vi "test_read-nmea-data2.vi"() -> ()   [LabVIEW 2019] (continued)
\t$GBGSV,2,2,06,33,62,220,31,34,,,33,1*41\n\t\n15:14:39.69\tF9P\t$GBGSV,1,1,03,11,48,133,,14,87,101,,33,62,220,,3*44\n\t\n15:14:39.71\tF9P\t$GNGLL,3723.60486,N,12656.97250,E,061441.00,A,A*77\n\t\n15:14:39.73\tF9P\t\t\n15:14:39.75\tF9P\t\t\n15:14:39.77\tF9P\t\t\n15:14:39.79\tF9P\t\t\n15:14:39.81\tF9P\t\t\n15:14:39.83\tF9P\t\t\n15:14:39.85\tF9P\t\t\n15:14:39.87\tF9P\t\t\n15:14:39.89\tF9P\t\t\n15:14:39.91\tF9P\t\t\n15:14:39.93\tF9P\t\t\n15:14:39.95\tF9P\t\t\n15:14:39.97\tF9P\t\t\n15:14:39.99\tF9P\t\t\n15:14:40.01\tF9P\t\t\n15:14:40.03\tF9P\t\t\n15:14:40.05\tF9P\t\t\n15:14:40.07\tF9P\t\t\n15:14:40.09\tF9P\t\t\n15:14:40.11\tF9P\t\t\n15:14:40.13\tF9P\t\t\n15:14:40.15\tF9P\t\t\n15:14:40.17\tF9P\t\t\n15:14:40.19\tF9P\t\t\n15:14:40.21\tF9P\t\t\n15:14:40.23\tF9P\t$GNRMC,061442.00,A,3723.60477,N,12656.97181,E,2.294,241.48,250720,,,A,V*0C\n\t\n15:14:40.25\tF9P\t$GNVTG,241.48,T,,M,2.294,N,4.248,K,A*2F\n\t\n15:14:40.27\tF9P\t$GNGGA,061442.00,3723.60477,N,12656.97181,E,1,12,0.66,44.9,M,18.5,M,,*76\n\t\n15:14:40.29\tF9P\t$GNGSA,A,3,12,06,19,05,17,09,04,02,,,,,1.17,0.66,0.97,1*09\n\t\n15:14:40.31\tF9P\t$GNGSA,A,3,85,70,71,84,,,,,,,,,1.17,0.66,0.97,2*0B\n\t\n15:14:40.33\tF9P\t$GNGSA,A,3,36,19,11,04,09,12,,,,,,,1.17,0.66,0.97,3*09\n\t\n15:14:40.35\tF9P\t$GNGSA,A,3,14,11,33,,,,,,,,,,1.17,0.66,0.97,4*08\n\t\n15:14:40.37\tF9P\t$GPGSV,3,1,09,02,55,320,33,04,17,043,38,05,38,248,35,06,64,050,28,1*6F\n\t\n15:14:40.39\tF9P\t$GPGSV,3,2,09,09,44,073,38,12,23,276,24,17,32,154,35,19,51,157,36,1*66\n\t\n15:14:40.41\tF9P\t$GPGSV,3,3,09,25,12,306,18,1*55\n\t\n15:14:40.43\tF9P\t$GPGSV,3,1,09,02,55,320,,04,17,043,26,05,38,248,25,06,64,050,24,6*6A\n\t\n15:14:40.45\tF9P\t$GPGSV,3,2,09,09,44,073,25,12,23,276,15,17,32,154,20,19,51,157,,6*6E\n\t\n15:14:40.47\tF9P\t$GPGSV,3,3,09,25,12,306,,6*5B\n\t\n15:14:40.49\tF9P\t$GLGSV,2,1,08,69,10,031,27,70,70,037,26,71,54,207,31,72,05,210,,1*79\n\t\n15:14:40.51\tF9P\t$GLGSV,2,2,08,77,01,324,,84,19,123,20,85,69,072,37,86,38,331,,1*75\n\t\n15:14:40.53\tF9P\t$GLGSV,2,1,08,69,10,031,21,70,70,037,,71,54,207,30,72,05,210,,3*78\n\t\n15:14:40.55\tF9P\t$GLGSV,2,2,08,77,01,324,,84,19,123,26,85,69,072,24,86,38,331,,3*73\n\t\n15:14:40.57\tF9P\t$GAGSV,2,1,08,02,08,296,11,04,67,115,24,09,33,193,27,11,72,001,24,7*7C\n\t\n15:14:40.59\tF9P\t$GAGSV,2,2,08,12,39,103,30,19,25,045,28,25,08,248,,36,27,309,19,7*74\n\t\n15:14:40.61\tF9P\t$GAGSV,2,1,08,02,08,296,,04,67,115,,09,33,193,,11,72,001,,2*7C\n\t\n15:14:40.63\tF9P\t$GAGSV,2,2,08,12,39,103,,19,25,045,,25,08,248,,36,27,309,,2*70\n\t\n15:14:40.65\tF9P\t$GBGSV,2,1,06,07,,,24,11,48,133,28,14,87,101,31,28,,,24,1*71\n\t\n15:14:40.67\tF9P\t$GBGSV,2,2,06,33,62,220,37,34,,,37,1*43\n\t\n15:14:40.69\tF9P\t$GBGSV,1,1,03,11,48,133,22,14,87,101,,33,62,220,,3*44\n\t\n15:14:40.71\tF9P\t$GNGLL,3723.60477,N,12656.97181,E,061442.00,A,A*75\n\t\n15:14:40.73\tF9P\t\t\n15:14:40.75\tF9P\t\t\n15:14:40.77\tF9P\t\t\n15:14:40.79\tF9P\t\t\n15:14:40.81\tF9P\t\t\n15:14:40.83\tF9P\t\t\n15:14:40.85\tF9P\t\t\n15:14:40.87\tF9P\t\t\n15:14:40.89\tF9P\t\t\n15:14:40.91\tF9P\t\t\n15:14:40.93\tF9P\t\t\n15:14:40.95\tF9P\t\t\n15:14:40.97\tF9P\t\t\n15:14:40.99\tF9P\t\t\n15:14:41.01\tF9P\t\t\n15:14:41.03\tF9P\t\t\n15:14:41.05\tF9P\t\t\n15:14:41.07\tF9P\t\t\n15:14:41.09\tF9P\t\t\n15:14:41.11\tF9P\t\t\n15:14:41.13\tF9P\t\t\n15:14:41.15\tF9P\t\t\n15:14:41.17\tF9P\t\t\n15:14:41.19\tF9P\t\t\n15:14:41.21\tF9P\t\t\n15:14:41.23\tF9P\t$GNRMC,061443.00,A,3723.60479,N,12656.97102,E,2.245,246.31,250720,,,A,V*0D\n\t\n15:14:41.25\tF9P\t$GNVTG,246.31,T,,M,2.245,N,4.157,K,A*27\n\t\n15:14:41.27\tF9P\t$GNGGA,061443.00,3723.60479,N,12656.97102,E,1,12,0.63,45.0,M,18.5,M,,*7F\n\t\n15:14:41.29\tF9P\t$GNGSA,A,3,12,06,19,05,17,09,04,02,,,,,1.14,0.63,0.95,1*0D\n\t\n15:14:41.31\tF9P\t$GNGSA,A,3,85,70,71,84,,,,,,,,,1.14,0.63,0.95,2*0F\n\t\n15:14:41.33\tF9P\t$GNGSA,A,3,36,19,11,04,09,12,,,,,,,1.14,0.63,0.95,3*0D\n\t\n15:14:41.35\tF9P\t$GNGSA,A,3,14,11,33,,,,,,,,,,1.14,0.63,0.95,4*0C\n\t\n15:14:41.37\tF9P\t$GPGSV,3,1,09,02,55,320,34,04,17,043,33,05,38,248,34,06,64,050,28,1*62\n\t\n15:14:41.39\tF9P\t$GPGSV,3,2,09,09,44,073,36,12,23,276,26,17,32,154,44,19,51,157,33,1*69\n\t\n15:14:41.41\tF9P\t$GPGSV,3,3,09,25,12,306,17,1*5A\n\t\n15:14:41.43\tF9P\t$GPGSV,3,1,09,02,55,320,,04,17,043,27,05,38,248,25,06,64,050,25,6*6A\n\t\n15:14:41.45\tF9P\t$GPGSV,3,2,09,09,44,073,25,12,23,276,14,17,32,154,21,19,51,157,,6*6E\n\t\n15:14:41.47\tF9P\t$GPGSV,3,3,09,25,12,306,,6*5B\n\t\n15:14:41.49\tF9P\t$GLGSV,2,1,08,69,10,031,32,70,70,037,27,71,54,207,35,72,05,210,,1*78\n\t\n15:14:41.51\tF9P\t$GLGSV,2,2,08,77,01,324,,84,19,123,19,85,69,072,35,86,38,331,,1*7D\n\t\n15:14:41.53\tF9P\t$GLGSV,2,1,08,69,10,031,20,70,70,037,,71,54,207,20,72,05,210,,3*78\n\t\n15:14:41.55\tF9P\t$GLGSV,2,2,08,77,01,324,,84,19,123,24,85,69,072,23,86,38,331,,3*76\n\t\n15:14:41.57\tF9P\t$GAGSV,2,1,08,02,08,296,10,04,67,115,26,09,33,193,32,11,72,001,24,7*7B\n\t\n15:14:41.59\tF9P\t$GAGSV,2,2,08,12,39,103,23,19,25,045,33,25,08,248,24,36,27,309,19,7*7A\n\t\n15:14:41.61\tF9P\t$GAGSV,2,1,08,02,08,296,,04,67,115,,09,33,193,,11,72,001,,2*7C\n\t\n15:14:41.63\tF9P\t$GAGSV,2,2,08,12,39,103,,19,25,045,,25,08,248,,36,27,309,,2*70\n\t\n15:14:41.65\tF9P\t$GBGSV,2,1,06,07,,,25,11,48,133,38,14,87,101,32,28,,,24,1*72\n\t\n15:14:41.67\tF9P\t$GBGSV,2,2,06,33,62,220,26,34,,,42,1*41\n\t\n15:14:41.69\tF9P\t$GBGSV,1,1,03,11,48,133,,14,87,101,,33,62,220,,3*44\n\t\n15:14:41.71\tF9P\t$GNGLL,3723.60479,N,12656.97102,E,061443.00,A,A*71\n\t\n15:14:41.73\tF9P\t\t\n15:14:41.75\tF9P\t\t\n15:14:41.77\tF9P\t\t\n15:14:41.79\tF9P\t\t\n15:14:41.81\tF9P\t\t\n15:14:41.83\tF9P\t\t\n15:14:41.85\tF9P\t\t\n15:14:41.87\tF9P\t\t\n15:14:41.89\tF9P\t\t\n15:14:41.91\tF9P\t\t\n15:14:41.93\tF9P\t\t\n15:14:41.95\tF9P\t\t\n15:14:41.97\tF9P\t\t\n15:14:41.99\tF9P\t\t\n15:14:42.01\tF9P\t\t\n15:14:42.03\tF9P\t\t\n15:14:42.05\tF9P\t\t\n15:14:42.07\tF9P\t\t\n15:14:42.09\tF9P\t\t\n15:14:42.11\tF9P\t\t\n15:14:42.13\tF9P\t\t\n15:14:42.15\tF9P\t\t\n15:14:42.17\tF9P\t\t\n15:14:42.19\tF9P\t\t\n15:14:42.21\tF9P\t\t\n15:14:42.23\tF9P\t$GNRMC,061444.00,A,3723.60478,N,12656.97021,E,2.480,246.00,250720,,,A,V*06\n\t\n15:14:42.25\tF9P\t$GNVTG,246.00,T,,M,2.480,N,4.594,K,A*21\n\t\n15:14:42.27\tF9P\t$GNGGA,061444.00,3723.60478,N,12656.97021,E,1,12,0.63,45.2,M,18.5,M,,*7B\n\t\n15:14:42.29\tF9P\t$GNGSA,A,3,12,06,19,05,17,09,04,02,,,,,1.14,0.63,0.95,1*0D\n\t\n15:14:42.31\tF9P\t$GNGSA,A,3,85,70,71,84,,,,,,,,,1.14,0.63,0.95,2*0F\n\t\n15:14:42.33\tF9P\t$GNGSA,A,3,36,19,11,04,09,12,,,,,,,1.14,0.63,0.95,3*0D\n\t\n15:14:42.35\tF9P\t$GNGSA,A,3,14,11,33,,,,,,,,,,1.14,0.63,0.95,4*0C\n\t\n15:14:42.37\tF9P\t$GPGSV,3,1,09,02,55,320,29,04,17,043,35,05,38,248,32,06,64,050,29,1*6F\n\t\n15:14:42.39\tF9P\t$GPGSV,3,2,09,09,44,073,36,12,23,276,26,17,32,154,42,19,51,157,33,1*6F\n\t\n15:14:42.41\tF9P\t$GPGSV,3,3,09,25,12,306,17,1*5A\n\t\n15:14:42.43\tF9P\t$GPGSV,3,1,09,02,55,320,,04,17,043,26,05,38,248,24,06,64,050,27,6*68\n\t\n15:14:42.45\tF9P\t$GPGSV,3,2,09,09,44,073,25,12,23,276,17,17,32,154,23,19,51,157,,6*6F\n\t\n15:14:42.47\tF9P\t$GPGSV,3,3,09,25,12,306,,6*5B\n\t\n15:14:42.49\tF9P\t$GLGSV,2,1,08,69,10,031,33,70,70,037,27,71,54,207,34,72,05,210,,1*78\n\t\n15:14:42.51\tF9P\t$GLGSV,2,2,08,77,01,324,,84,19,123,20,85,69,072,31,86,38,331,,1*73\n\t\n15:14:42.53\tF9P\t$GLGSV,2,1,08,69,10,031,20,70,70,037,,71,54,207,22,72,05,210,,3*7A\n\t\n15:14:42.55\tF9P\t$GLGSV,2,2,08,77,01,324,,84,19,123,30,85,69,072,24,86,38,331,,3*74\n\t\n15:14:42.57\tF9P\t$GAGSV,2,1,08,02,08,296,09,04,67,115,31,09,33,193,32,11,72,001,24,7*75\n\t\n15:14:42.59\tF9P\t$GAGSV,2,2,08,12,39,103,23,19,25,045,35,25,08,248,23,36,27,309,20,7*71\n\t\n15:14:42.61\tF9P\t$GAGSV,2,1,08,02,08,296,,04,67,115,,09,33,193,,11,72,001,,2*7C\n\t\n15:14:42.63\tF9P\t$GAGSV,2,2,08,12,39,103,,19,25,045,,25,08,248,,36,27,309,,2*70\n\t\n15:14:42.65\tF9P\t$GBGSV,2,1,06,07,,,25,11,48,133,39,14,87,101,27,28,,,26,1*75\n\t\n15:14:42.67\tF9P\t$GBGSV,2,2,06,33,62,220,31,34,,,46,1*43\n\t\n15:14:42.69\tF9P\t$GBGSV,1,1,03,11,48,133,24,14,87,101,,33,62,220,,3*42\n\t\n15:14:42.71\tF9P\t$GNGLL,3723.60478,N,12656.97021,E,061444.00,A,A*77\n\t\n15:14:42.73\tF9P\t\t\n15:14:42.75\tF9P\t\t\n15:14:42.77\tF9P\t\t\n15:14:42.79\tF9P\t\t\n15:14:42.81\tF9P\t\t\n15:14:42.83\tF9P\t\t\n15:14:42.85\tF9P\t\t\n15:14:42.87\tF9P\t\t\n15:14:42.89\tF9P\t\t\n15:14:42.91\tF9P\t\t\n15:14:42.93\tF9P\t\t\n15:14:42.95\tF9P\t\t\n15:14:42.97\tF9P\t\t\n15:14:42.99\tF9P\t\t\n15:14:43.01\tF9P\t\t\n15:14:43.03\tF9P\t\t\n15:14:43.05\tF9P\t\t\n15:14:43.07\tF9P\t\t\n15:14:43.09\tF9P\t\t\n15:14:43.11\tF9P\t\t\n15:14:43.13\tF9P\t\t\n15:14:43.15\tF9P\t\t\n15:14:43.17\tF9P\t\t\n15:14:43.19\tF9P\t\t\n15:14:43.21\tF9P\t\t\n15:14:43.23\tF9P\t$GNRMC,061445.00,A,3723.60468,N,12656.96939,E,2.508,244.25,250720,,,A,V*03\n\t\n15:14:43.25\tF9P\t$GNVTG,244.25,T,,M,2.508,N,4.645,K,A*2A\n\t\n15:14:43.27\tF9P\t$GNGGA,061445.00,3723.60468,N,12656.96939,E,1,12,0.66,45.7,M,18.5,M,,*7A\n\t\n15:14:43.29\tF9P\t$GNGSA,A,3,12,06,19,05,17,09,04,02,,,,,1.17,0.66,0.97,1*09\n\t\n15:14:43.31\tF9P\t$GNGSA,A,3,85,70,71,84,,,,,,,,,1.17,0.66,0.97,2*0B\n\t\n15:14:43.33\tF9P\t$GNGSA,A,3,36,19,11,04,09,12,,,,,,,1.17,0.66,0.97,3*09\n\t\n15:14:43.35\tF9P\t$GNGSA,A,3,14,11,33,,,,,,,,,,1.17,0.66,0.97,4*08\n\t\n15:14:43.37\tF9P\t$GPGSV,3,1,09,02,55,320,30,04,17,043,35,05,38,248,35,06,64,050,36,1*6E\n\t\n15:14:43.39\tF9P\t$GPGSV,3,2,09,09,44,073,37,12,23,276,26,17,32,154,28,19,51,157,28,1*68\n\t\n15:14:43.41\tF9P\t$GPGSV,3,3,09,25,12,306,16,1*5B\n\t\n15:14:43.43\tF9P\t$GPGSV,3,1,09,02,55,320,,04,17,043,25,05,38,248,24,06,64,050,27,6*6B\n\t\n15:14:43.45\tF9P\t$GPGSV,3,2,09,09,44,073,26,12,23,276,18,17,32,154,22,19,51,157,,6*62\n\t\n15:14:43.47\tF9P\t$GPGSV,3,3,09,25,12,306,,6*5B\n\t\n15:14:43.49\tF9P\t$GLGSV,2,1,08,69,10,031,29,70,70,037,27,71,54,207,39,72,05,210,,1*7E\n\t\n15:14:43.51\tF9P\t$GLGSV,2,2,08,77,01,324,,84,19,123,21,85,69,072,34,86,38,331,,1*77\n\t\n15:14:43.53\tF9P\t$GLGSV,2,1,08,69,10,031,20,70,70,037,,71,54,207,24,72,05,210,,3*7C\n\t\n15:14:43.55\tF9P\t$GLGSV,2,2,08,77,01,324,,84,19,123,25,85,69,072,26,86,38,331,,3*72\n\t\n15:14:43.57\tF9P\t$GAGSV,2,1,08,02,08,296,09,04,67,115,33,09,33,193,26,11,72,001,24,7*72\n\t\n15:14:43.59\tF9P\t$GAGSV,2,2,08,12,39,103,31,19,25,045,26,25,08,248,21,36,27,309,20,7*72\n\t\n15:14:43.61\tF9P\t$GAGSV,2,1,08,02,08,296,,04,67,115,21,09,33,193,,11,72,001,,2*7F\n\t\n15:14:43.63\tF9P\t$GAGSV,2,2,08,12,39,103,,19,25,045,,25,08,248,,36,27,309,,2*70\n\t\n15:14:43.65\tF9P\t$GBGSV,2,1,06,07,,,25,11,48,133,39,14,87,101,27,28,,,25,1*76\n\t\n15:14:43.67\tF9P\t$GBGSV,2,2,06,33,62,220,34,34,,,37,1*40\n\t\n15:14:43.69\tF9P\t$GBGSV,1,1,03,11,48,133,26,14,87,101,29,33,62,220,,3*4B\n\t\n15:14:43.71\tF9P\t$GNGLL,3723.60468,N,12656.96939,E,061445.00,A,A*76\n\t\n15:14:43.73\tF9P\t\t\n15:14:43.75\tF9P\t\t\n15:14:43.77\tF9P\t\t\n15:14:43.79\tF9P\t\t\n15:14:43.81\tF9P\t\t\n15:14:43.83\tF9P\t\t\n15:14:43.85\tF9P\t\t\n15:14:43.87\tF9P\t\t\n15:14:43.89\tF9P\t\t\n15:14:43.91\tF9P\t\t\n15:14:43.93\tF9P\t\t\n15:14:43.95\tF9P\t\t\n15:14:43.97\tF9P\t\t\n15:14:43.99\tF9P\t\t\n15:14:44.01\tF9P\t\t\n15:14:44.03\tF9P\t\t\n15:14:44.05\tF9P\t\t\n15:14:44.07\tF9P\t\t\n15:14:44.09\tF9P\t\t\n15:14:44.11\tF9P\t\t\n15:14:44.13\tF9P\t\t\n15:14:44.15\tF9P\t\t\n15:14:44.17\tF9P\t\t\n15:14:44.19\tF9P\t\t\n15:14:44.21\tF9P\t\t\n15:14:44.23\tF9P\t$GNRMC,061446.00,A,3723.60454,N,12656.96856,E,2.232,243.16,250720,,,A,V*0E\n\t\n15:14:44.25\tF9P\t$GNVTG,243.16,T,,M,2.232,N,4.135,K,A*23\n\t\n15:14:44.27\tF9P\t$GNGGA,061446.00,3723.60454,N,12656.96856,E,1,12,0.66,45.7,M,18.5,M,,*7E\n\t\n15:14:44.29\tF9P\t$GNGSA,A,3,12,06,19,05,17,09,04,02,,,,,1.17,0.66,0.97,1*09\n\t\n15:14:44.31\tF9P\t$GNGSA,A,3,85,70,71,84,,,,,,,,,1.17,0.66,0.97,2*0B\n\t\n15:14:44.33\tF9P\t$GNGSA,A,3,36,19,11,04,09,12,,,,,,,1.17,0.66,0.97,3*09\n\t\n15:14:44.35\tF9P\t$GNGSA,A,3,14,11,33,,,,,,,,,,1.17,0.66,0.97,4*08\n\t\n15:14:44.37\tF9P\t$GPGSV,3,1,09,02,56,320,29,04,17,043,30,05,38,248,35,06,64,050,40,1*61\n\t\n15:14:44.39\tF9P\t$GPGSV,3,2,09,09,44,073,33,12,23,276,25,17,32,154,33,19,51,157,36,1*6A\n\t\n15:14:44.41\tF9P\t$GPGSV,3,3,09,25,12,306,16,1*5B\n\t\n15:14:44.43\tF9P\t$GPGSV,3,1,09,02,56,320,,04,17,043,24,05,38,248,25,06,64,050,27,6*68\n\t\n15:14:44.45\tF9P\t$GPGSV,3,2,09,09,44,073,25,12,23,276,17,17,32,154,20,19,51,157,,6*6C\n\t\n15:14:44.47\tF9P\t$GPGSV,3,3,09,25,12,306,,6*5B\n\t\n15:14:44.49\tF9P\t$GLGSV,2,1,08,69,10,031,31,70,70,037,29,71,54,207,36,72,05,210,,1*76\n\t\n15:14:44.51\tF9P\t$GLGSV,2,2,08,77,01,324,,84,19,123,22,85,69,072,28,86,38,331,,1*79\n\t\n15:14:44.53\tF9P\t$GLGSV,2,1,08,69,10,031,19,70,70,037,,71,54,207,24,72,05,210,,3*76\n\t\n15:14:44.55\tF9P\t$GLGSV,2,2,08,77,01,324,,84,19,123,31,85,69,072,26,86,38,331,,3*77\n\t\n15:14:44.57\tF9P\t$GAGSV,2,1,08,02,08,296,10,04,67,115,36,09,33,193,28,11,72,001,24,7*71\n\t\n15:14:44.59\tF9P\t$GAGSV,2,2,08,12,39,103,30,19,25,045,31,25,08,248,21,36,27,309,19,7*7F\n\t\n15:14:44.61\tF9P\t$GAGSV,2,1,08,02,08,296,,04,67,115,22,09,33,193,,11,72,001,,2*7C\n\t\n15:14:44.63\tF9P\t$GAGSV,2,2,08,12,39,103,,19,25,045,,25,08,248,,36,27,309,,2*70\n\t\n15:14:44.65\tF9P\t$GBGSV,2,1,06,07,,,24,11,48,133,41,14,87,101,28,28,,,24,1*76\n\t\n15:14:44.67\tF9P\t$GBGSV,2,2,06,33,62,220,23,34,,,32,1*43\n\t\n15:14:44.69\tF9P\t$GBGSV,1,1,03,11,48,133,25,14,87,101,,33,62,220,,3*43\n\t\n15:14:44.71\tF9P\t$GNGLL,3723.60454,N,12656.96856,E,061446.00,A,A*72\n\t\n15:14:44.73\tF9P\t\t\n15:14:44.75\tF9P\t\t\n15:14:44.77\tF9P\t\t\n15:14:44.79\tF9P\t\t\n15:14:44.81\tF9P\t\t\n15:14:44.84\tF9P\t\t\n15:14:44.86\tF9P\t\t\n15:14:44.88\tF9P\t\t\n15:14:44.90\tF9P\t\t\n15:14:44.92\tF9P\t\t\n15:14:44.94\tF9P\t\t\n15:14:44.96\tF9P\t\t\n15:14:44.98\tF9P\t\t\n15:14:45.00\tF9P\t\t\n15:14:45.02\tF9P\t\t\n15:14:45.04\tF9P\t\t\n15:14:45.06\tF9P\t\t\n15:14:45.08\tF9P\t\t\n15:14:45.10\tF9P\t\t\n15:14:45.12\tF9P\t\t\n15:14:45.14\tF9P\t\t\n15:14:45.16\tF9P\t\t\n15:14:45.18\tF9P\t\t\n15:14:45.20\tF9P\t\t\n15:14:45.22\tF9P\t\t\n15:14:45.24\tF9P\t$GNRMC,061447.00,A,3723.60450,N,12656.96767,E,2.336,245.60,250720,,,A,V*04\n\t\n15:14:45.26\tF9P\t$GNVTG,245.60,T,,M,2.336,N,4.325,K,A*22\n\t\n15:14:45.28\tF9P\t$GNGGA,061447.00,3723.60450,N,12656.96767,E,1,12,0.63,46.1,M,18.5,M,,*76\n\t\n15:14:45.30\tF9P\t$GNGSA,A,3,12,06,19,05,17,09,04,02,,,,,1.14,0.63,0.95,1*0D\n\t\n15:14:45.32\tF9P\t$GNGSA,A,3,85,70,71,84,,,,,,,,,1.14,0.63,0.95,2*0F\n\t\n15:14:45.34\tF9P\t$GNGSA,A,3,36,19,11,04,09,12,,,,,,,1.14,0.63,0.95,3*0D\n\t\n15:14:45.36\tF9P\t$GNGSA,A,3,14,11,33,,,,,,,,,,1.14,0.63,0.95,4*0C\n\t\n15:14:45.38\tF9P\t$GPGSV,3,1,09,02,56,320,25,04,17,043,37,05,38,248,38,06,64,050,38,1*68\n\t\n15:14:45.40\tF9P\t$GPGSV,3,2,09,09,44,073,37,12,23,276,25,17,32,154,27,19,51,157,28,1*64\n\t\n15:14:45.42\tF9P\t$GPGSV,3,3,09,25,12,306,16,1*5B\n\t\n15:14:45.44\tF9P\t$GPGSV,3,1,09,02,56,320,,04,17,043,26,05,38,248,25,06,64,050,27,6*6A\n\t\n15:14:45.46\tF9P\t$GPGSV,3,2,09,09,44,073,25,12,23,276,18,17,32,154,18,19,51,157,,6*68\n\t\n15:14:45.48\tF9P\t$GPGSV,3,3,09,25,12,306,,6*5B\n\t\n15:14:45.50\tF9P\t$GLGSV,2,1,08,69,10,031,26,70,70,037,29,71,54,207,34,72,05,210,,1*72\n\t\n15:14:45.52\tF9P\t$GLGSV,2,2,08,77,01,324,,84,19,123,22,85,69,072,31,86,38,331,,1*71\n\t\n15:14:45.54\tF9P\t$GLGSV,2,1,08,69,10,031,21,70,70,037,,71,54,207,24,72,05,210,,3*7D\n\t\n15:14:45.56\tF9P\t$GLGSV,2,2,08,77,01,324,,84,19,123,30,85,69,072,26,86,38,331,,3*76\n\t\n15:14:45.58\tF9P\t$GAGSV,2,1,08,02,08,296,10,04,67,115,37,09,33,193,33,11,72,001,25,7*7B\n\t\n15:14:45.60\tF9P\t$GAGSV,2,2,08,12,39,103,29,19,25,045,34,25,08,248,21,36,27,309,19,7*72\n\t\n15:14:45.62\tF9P\t$GAGSV,2,1,08,02,08,296,,04,67,115,22,09,33,193,,11,72,001,,2*7C\n\t\n15:14:45.64\tF9P\t$GAGSV,2,2,08,12,39,103,,19,25,045,,25,08,248,,36,27,309,,2*70\n\t\n15:14:45.66\tF9P\t$GBGSV,2,1,06,07,,,25,11,48,133,40,14,87,101,26,28,,,25,1*79\n\t\n15:14:45.68\tF9P\t$GBGSV,2,2,06,33,62,220,29,34,,,31,1*4A\n\t\n15:14:45.70\tF9P\t$GBGSV,1,1,03,11,48,133,25,14,87,101,,33,62,220,,3*43\n\t\n15:14:45.72\tF9P\t$GNGLL,3723.60450,N,12656.96767,E,061447.00,A,A*7A\n\t\n15:14:45.74\tF9P\t\t\n15:14:45.76\tF9P\t\t\n15:14:45.78\tF9P\t\t\n15:14:45.80\tF9P\t\t\n15:14:45.82\tF9P\t\t\n15:14:45.84\tF9P\t\t\n15:14:45.86\tF9P\t\t\n15:14:45.88\tF9P\t\t\n15:14:45.90\tF9P\t\t\n15:14:45.92\tF9P\t\t\n15:14:45.94\tF9P\t\t\n15:14:45.96\tF9P\t\t\n15:14:45.98\tF9P\t\t\n15:14:46.00\tF9P\t\t\n15:14:46.02\tF9P\t\t\n15:14:46.04\tF9P\t\t\n15:14:46.06\tF9P\t\t\n15:14:46.08\tF9P\t\t\n15:14:46.10\tF9P\t\t\n15:14:46.12\tF9P\t\t\n15:14:46.14\tF9P\t\t\n15:14:46.16\tF9P\t\t\n15:14:46.18\tF9P\t\t\n15:14:46.20\tF9P\t\t\n15:14:46.22\tF9P\t\t\n15:14:46.24\tF9P\t$GNRMC,061448.00,A,3723.60435,N,12656.96701,E,2.322,243.14,250720,,,A,V*08\n\t\n15:14:46.26\tF9P\t$GNVTG,243.14,T,,M,2.322,N,4.301,K,A*24\n\t\n15:14:46.28\tF9P\t$GNGGA,061448.00,3723.60435,N,12656.96701,E,1,12,0.63,46.2,M,18.5,M,,*79\n\t\n15:14:46.30\tF9P\t$GNGSA,A,3,12,06,19,05,17,09,04,02,,,,,1.14,0.63,0.95,1*0D\n\t\n15:14:46.32\tF9P\t$GNGSA,A,3,85,70,71,84,,,,,,,,,1.14,0.63,0.95,2*0F\n\t\n15:14:46.34\tF9P\t$GNGSA,A,3,36,19,11,04,09,12,,,,,,,1.14,0.63,0.95,3*0D\n\t\n15:14:46.36\tF9P\t$GNGSA,A,3,14,11,33,,,,,,,,,,1.14,0.63,0.95,4*0C\n\t\n15:14:46.38\tF9P\t$GPGSV,3,1,09,02,56,320,23,04,17,043,35,05,38,248,36,06,64,050,31,1*6B\n\t\n15:14:46.40\tF9P\t$GPGSV,3,2,09,09,44,073,30,12,23,276,25,17,32,154,30,19,51,157,27,1*6A\n\t\n15:14:46.42\tF9P\t$GPGSV,3,3,09,25,12,306,15,1*58\n\t\n15:14:46.44\tF9P\t$GPGSV,3,1,09,02,56,320,,04,17,043,24,05,38,248,27,06,64,050,27,6*6A\n\t\n15:14:46.46\tF9P\t$GPGSV,3,2,09,09,44,073,26,12,23,276,17,17,32,154,16,19,51,157,,6*6A\n\t\n15:14:46.48\tF9P\t$GPGSV,3,3,09,25,12,306,,6*5B\n\t\n15:14:46.50\tF9P\t$GLGSV,2,1,08,69,10,031,27,70,70,037,28,71,54,207,38,72,05,210,,1*7E\n\t\n15:14:46.52\tF9P\t$GLGSV,2,2,08,77,01,324,,84,19,123,21,85,69,072,30,86,38,331,,1*73\n\t\n15:14:46.54\tF9P\t$GLGSV,2,1,08,69,10,031,21,70,70,037,,71,54,207,24,72,05,210,,3*7D\n\t\n15:14:46.56\tF9P\t$GLGSV,2,2,08,77,01,324,,84,19,123,28,85,69,072,25,86,38,331,,3*7C\n\t\n15:14:46.58\tF9P\t$GAGSV,2,1,08,02,08,296,09,04,67,115,38,09,33,193,34,11,72,001,24,7*7A\n\t\n15:14:46.60\tF9P\t$GAGSV,2,2,08,12,39,103,28,19,25,045,34,25,08,248,21,36,27,309,18,7*72\n\t\n15:14:46.62\tF9P\t$GAGSV,2,1,08,02,08,296,,04,67,115,23,09,33,193,,11,72,001,,2*7D\n\t\n15:14:46.64\tF9P\t$GAGSV,2,2,08,12,39,103,,19,25,045,,25,08,248,,36,27,309,,2*70\n\t\n15:14:46.66\tF9P\t$GBGSV,2,1,06,07,,,24,11,48,133,37,14,87,101,26,28,,,25,1*78\n\t\n15:14:46.68\tF9P\t$GBGSV,2,2,06,33,62,220,28,34,,,38,1*42\n\t\n15:14:46.70\tF9P\t$GBGSV,1,1,03,11,48,133,25,14,87,101,,33,62,220,,3*43\n\t\n15:14:46.72\tF9P\t$GNGLL,3723.60435,N,12656.96701,E,061448.00,A,A*76\n\t\n15:14:46.74\tF9P\t\t\n15:14:46.76\tF9P\t\t\n15:14:46.78\tF9P\t\t\n15:14:46.80\tF9P\t\t\n15:14:46.82\tF9P\t\t\n15:14:46.84\tF9P\t\t\n15:14:46.86\tF9P\t\t\n15:14:46.88\tF9P\t\t\n15:14:46.90\tF9P\t\t\n15:14:46.92\tF9P\t\t\n15:14:46.94\tF9P\t\t\n15:14:46.96\tF9P\t\t\n15:14:46.98\tF9P\t\t\n15:14:47.00\tF9P\t\t\n15:14:47.02\tF9P\t\t\n15:14:47.04\tF9P\t\t\n15:14:47.06\tF9P\t\t\n15:14:47.08\tF9P\t\t\n15:14:47.10\tF9P\t\t\n15:14:47.12\tF9P\t\t\n15:14:47.14\tF9P\t\t\n15:14:47.16\tF9P\t\t\n15:14:47.18\tF9P\t\t\n15:14:47.20\tF9P\t\t\n15:14:47.22\tF9P\t\t\n15:14:47.24\tF9P\t$GNRMC,061449.00,A,3723.60420,N,12656.96638,E,2.502,240.62,250720,,,A,V*00\n\t\n15:14:47.26\tF9P\t$GNVTG,240.62,T,,M,2.502,N,4.634,K,A*21\n\t\n15:14:47.28\tF9P\t$GNGGA,061449.00,3723.60420,N,12656.96638,E,1,12,0.63,46.3,M,18.5,M,,*76\n\t\n15:14:47.30\tF9P\t$GNGSA,A,3,12,06,19,05,17,09,04,02,,,,,1.14,0.63,0.95,1*0D\n\t\n15:14:47.32\tF9P\t$GNGSA,A,3,85,70,71,84,,,,,,,,,1.14,0.63,0.95,2*0F\n\t\n15:14:47.34\tF9P\t$GNGSA,A,3,36,19,11,04,09,12,,,,,,,1.14,0.63,0.95,3*0D\n\t\n15:14:47.36\tF9P\t$GNGSA,A,3,14,11,33,,,,,,,,,,1.14,0.63,0.95,4*0C\n\t\n15:14:47.38\tF9P\t$GPGSV,3,1,09,02,56,320,24,04,17,043,33,05,38,248,32,06,64,050,35,1*6A\n\t\n15:14:47.40\tF9P\t$GPGSV,3,2,09,09,44,073,36,12,23,276,25,17,32,154,26,19,51,157,27,1*6B\n\t\n15:14:47.42\tF9P\t$GPGSV,3,3,09,25,12,306,16,1*5B\n\t\n15:14:47.44\tF9P\t$GPGSV,3,1,09,02,56,320,,04,17,043,22,05,38,248,27,06,64,050,27,6*6C\n\t\n15:14:47.46\tF9P\t$GPGSV,3,2,09,09,44,073,27,12,23,276,17,17,
